vi "Check_Invalid_Characters_In_Name.vi"(6 "AB_Destination":refnum<class "AB_Destination.lvclass">, 7 "AB_Source in":refnum<class "AB_Source.lvclass">, 8 "error in (no error)":errorcluster, 9 "update name":bool, 10 "file name in":string, 11 "Build in":refnum<class "AB_PackedLibrary.lvclass">) -> (0 "error out":errorcluster, 1 "updated":bool, 2 "file name out":string, 3 "Build out":refnum<class "AB_PackedLibrary.lvclass">, 5 "AB_Source out":refnum<class "AB_Source.lvclass">)   [LabVIEW 2020, in "AB_PackedLibrary.lvclass"]
uses:
  <vilib>/AppBuilder/AB_Classes/PackedLib/AB_PackedLibrary.lvclass
  <vilib>/AppBuilder/AB_Classes/Destination/AB_Destination.lvclass
  <vilib>/AppBuilder/AB_Classes/Source/AB_Source.lvclass
  <vilib>/AppBuilder/AB_Classes/TargetFile/AB_Targetfile.lvclass
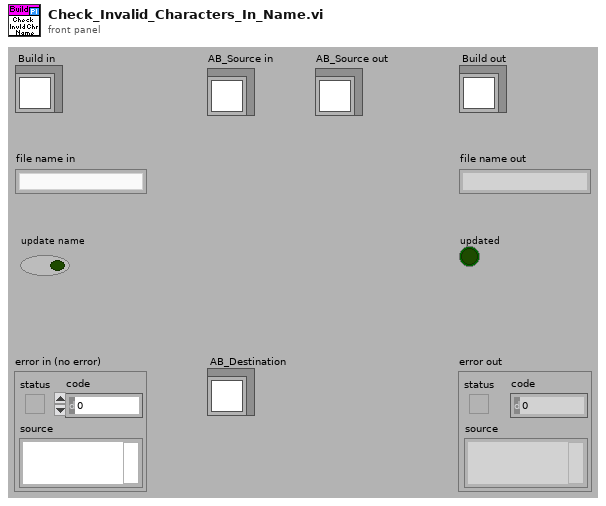
[diagram p1: front panel]
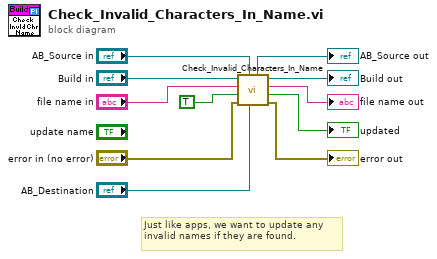
[diagram p0: block diagram]
diagram:
  # "Just like apps, we want to update any invalid names if they are found."
  n1 = call-parent "Check_Invalid_Characters_In_Name.vi"("AB_Destination in"="AB_Destination", "AB_Source in"="AB_Source in", "error in (no error)"="error in (no error)", "update name"=TRUE, "file name in"="file name in", "Build in"="Build in") -> ("error out"=→"error out":errorcluster, "updated"=→"updated":bool, "file name out"=→"file name out":string, "Build out"=→"Build out":refnum<class "AB_PackedLibrary.lvclass">, "AB_Source out"=→"AB_Source out":refnum<class "AB_Source.lvclass">)  [unwired: 1 out]
